vi "Controller Load Filter Coefficients.vi"(8 "error in (no error)":errorcluster, 11 "Coefficients":fxp<+/-,20,2>[](array[numeric])) -> (0 "error out":errorcluster, 3 "All coefficients loaded?":bool)   [LabVIEW 2011, in "Controller VIs.lvlib"]
uses:
  Controller VIs.lvlib
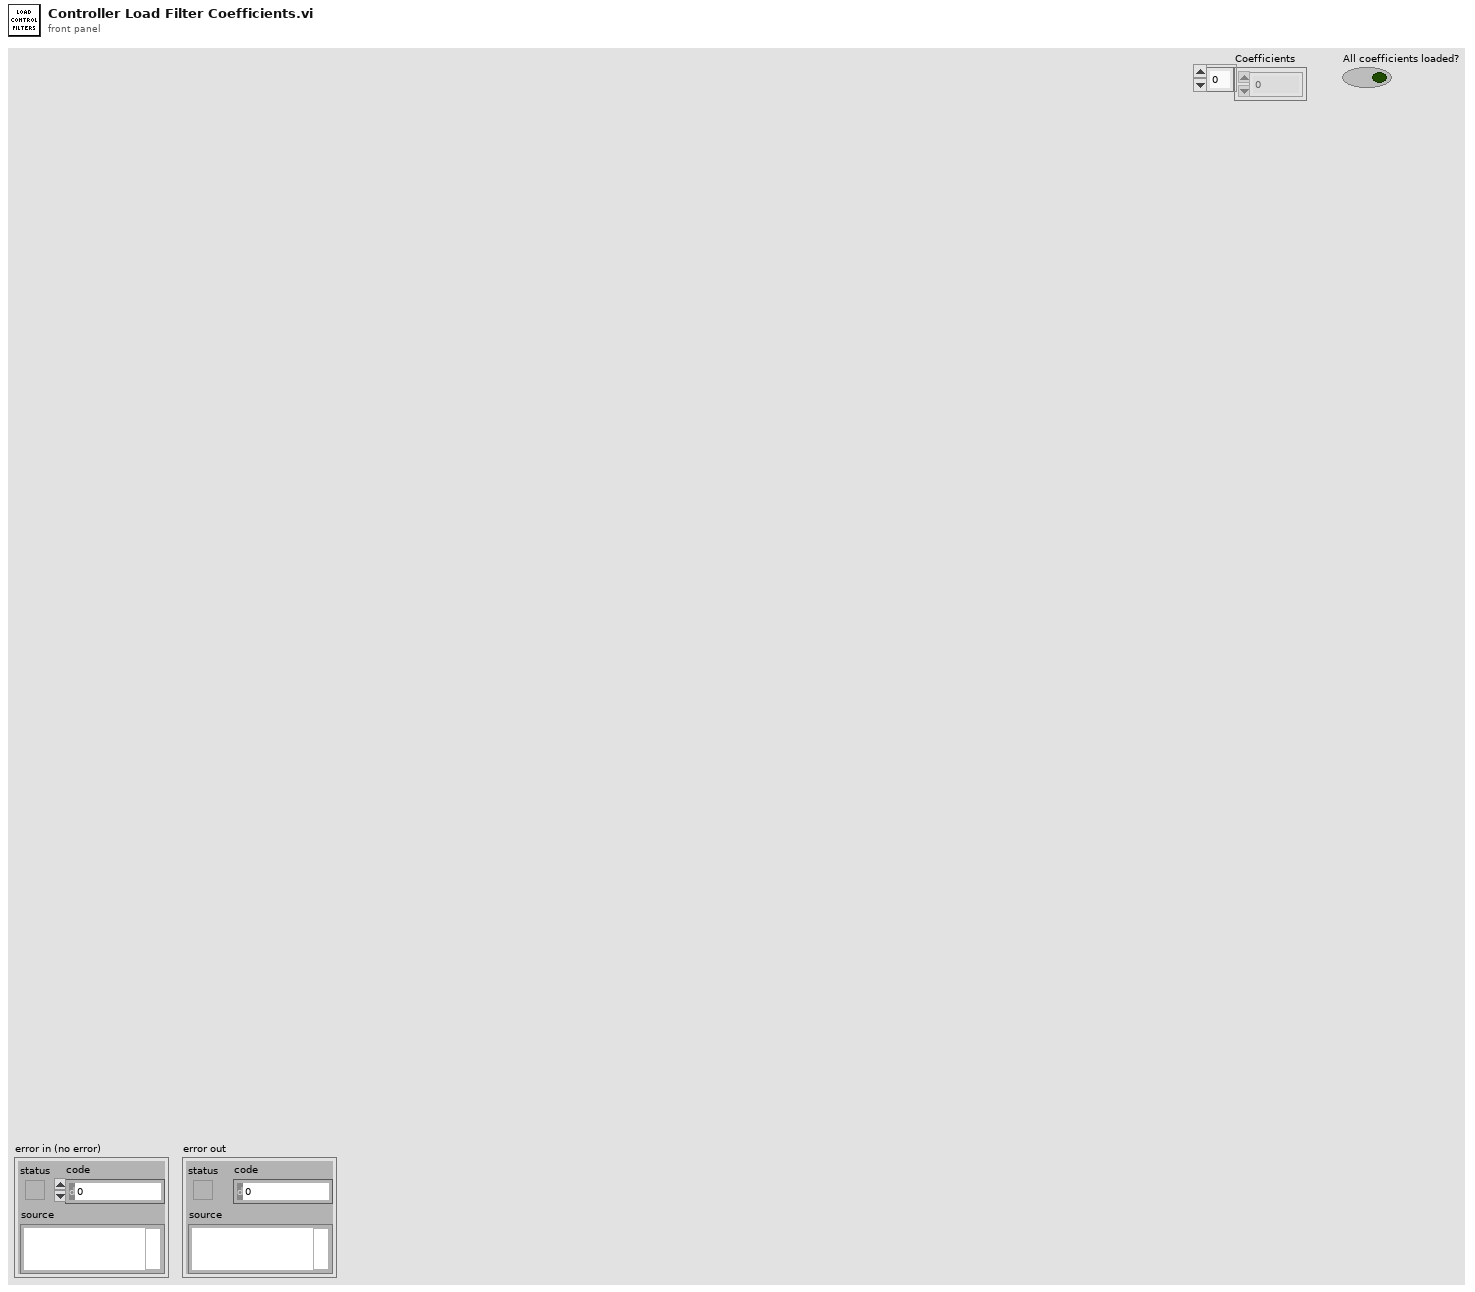
[diagram p1: front panel]
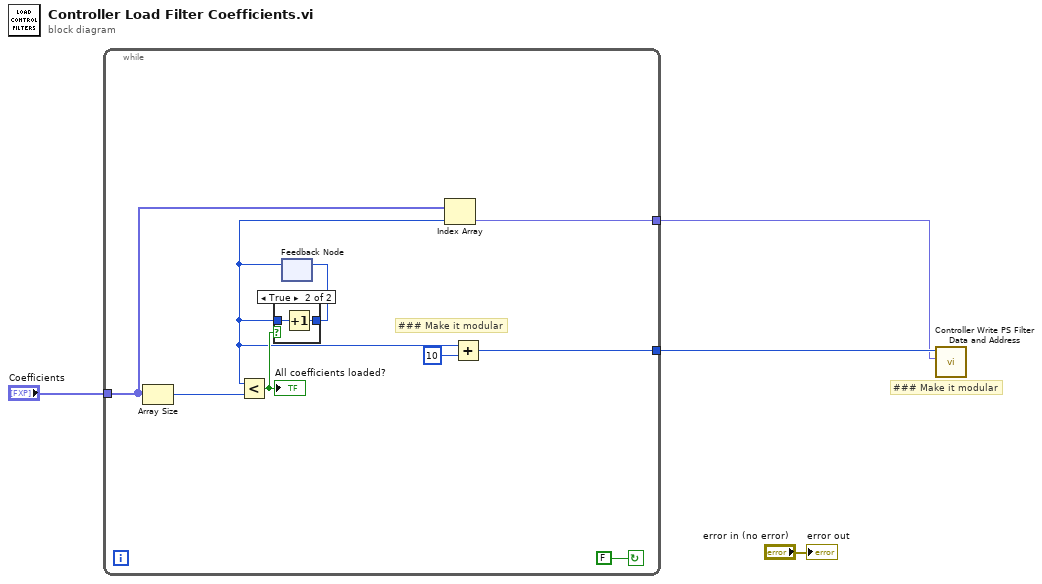
[diagram p0: block diagram]
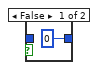
[diagram p2: hidden frame]
diagram:
  # "### Make it modular"
  n1 = while {
    tunnel: "Coefficients" -> [w5]
    tunnel: [w9] -> w2
    tunnel: [w7] -> w1
    stop <- FALSE continue-if-true
    # "### Make it modular"
    n2 = Array Size(array=w5) -> (size(s)=w8:i32)
    n3 = feedback #1() -> (w6:u8)  [unwired: 1 in]
    n4 = Less?(x=w6, y=w8) -> (x < y?=w13:bool)
    "All coefficients loaded?" <- w13
    n5 = case shown="True" w13 {
      tunnel: w6 -> [_ w16]
      tunnel: [u8 0 w15] -> w12
      frame False {
      }
      frame True {
        n6 = Increment(x=w16) -> (x+1=w15:u8)
      }
    }
    n7 = feedback-in #1(w12) -> ()
    n8 = Index Array(array=w5, index=w6) -> (element=w7:fxp<+/-,20,2>)
    n9 = Add(x=w6, y=u8 10) -> (x+y=w9:u8)
  }
  n10 = call "Controller Write PS Filter Data and Address.vi"("Data"=w1, "Address"=w2) -> ()  [unwired: 10 in]
  "error out" <- "error in (no error)"
